vi "Motor.vi"(2 "DESV-IN":bool, 3 "BrickReference in":T1) -> (0 "DESV-OUT":bool, 1 "BrickReference out":T1)   [LabVIEW 2015]
uses:
  <vilib>/NXT/Subs/LVHSConnector.ctl
  <vilib>/NXT/LegoClasses/BrickReference/BrickReference.lvclass
  <vilib>/NXT/Block Support/NXT_OutputPort.ctl
  <vilib>/NXT/Subs/MotorOutput.ctl
  <vilib>/NXT/NXTIO Xnodes/NXTIONodeSubVIs/NXTMotorSteeringOn.vi
  <vilib>/NXT/Dual Mode Library/Sound/Tone.vi
  <vilib>/NXT/NXTIO Xnodes/AddressXNode/NXTIOAddress.xnode
  <vilib>/NXT/NXTIO Xnodes/NXTIOXNode/NXTIO.xnode
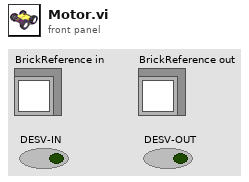
[diagram p1: front panel]
types:
  T1 = typedef "LVHSConnector.ctl" = refnum<class "BrickReference.lvclass">
  T2 = typedef "NXT_OutputPort.ctl" = u8
  T3 = typedef "MotorOutput.ctl" = u8
  T4 = cluster{"PowerLeft":i32, "RotationLeft(Degrees)":i32, "PortLeft":T3}
  T5 = cluster{"PowerRight":i32, "RotationRight(Degrees)":i32, "PortRight":T3}
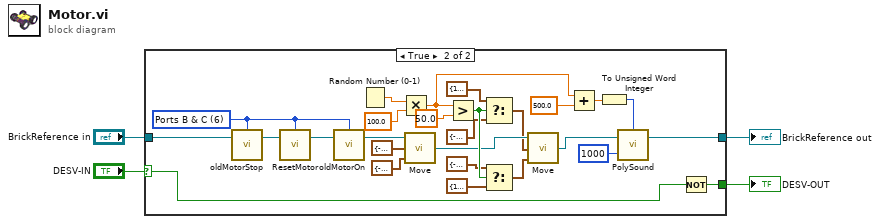
[diagram p0: block diagram]
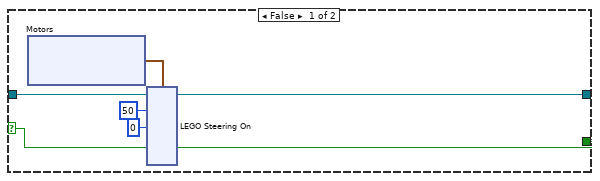
[diagram p2: hidden frame]
diagram:
  n1 = case shown="True" "DESV-IN" {
    selector: "DESV-IN" -> [w6 w22]
    tunnel: "BrickReference in" -> [w10 w46]
    tunnel: [w6 w21] -> w3
    tunnel: [w5 w20] -> w4
    frame False {
      n2 = xnode "Motors"() -> ("Motor"=w9:cluster{"Port":T2, "Port":T2})
      n3 = xnode "LEGO Steering On"("Steering 1"=0, "Power 1"=50, "Motors"=w9, "NXT/EV3"=w10) -> ("NXT/EV3"=w5:T1)
    }
    frame True {
      w43 = T3 6 items=["Port A"=0, "Port B"=1, "Port C"=2, "Ports A & B"=4, "Ports A & C"=5, "Ports B & C"=6, "All Ports"=3] ("Output Port (All Ports)")
      n4 = call <vilib>:"oldMotorStop.vi"("NXT/EV3"=w46, "Output Port (All Ports)"=w43) -> ("NXT/EV3"=w45:T1)  [unwired: 2 in]
      n5 = call <vilib>:"ResetMotor.vi"("NXT/EV3"=w45, "Port (All Ports)"=w43) -> ("NXT/EV3"=w44:T1)  [unwired: 2 in]
      n6 = call <vilib>:"oldMotorOn.vi"("NXT/EV3"=w44, "Output Port (All Ports)"=w43) -> ("NXT/EV3"=w42:T1)  [unwired: 2 in]
      n7 = Random Number (0-1)() -> (number: 0 to 1=w38:dbl)
      n8 = Multiply(x=w38, y=100.0) -> (x*y=w27:dbl)
      n9 = call "Move.vi"("Right"=T4 {"PowerLeft"=-100, "RotationLeft(Degrees)"=-360, "PortLeft"=1} ("Left"), "Left"=T5 {"PowerRight"=-100, "RotationRight(Degrees)"=-360, "PortRight"=2} ("Right"), "BrickReference in"=w42) -> ("BrickReference out"=w31:T1)
      n10 = Greater?(x=w27, y=50.0) -> (0:w36:bool)
      n11 = Select(t=T5 {"PowerRight"=100, "RotationRight(Degrees)"=360, "PortRight"=2} ("Right"), s=w36, f=T5 {"PowerRight"=-100, "RotationRight(Degrees)"=-360, "PortRight"=2} ("Right")) -> (s? t:f=w29:T5)
      n12 = Select(t=T4 {"PowerLeft"=-100, "RotationLeft(Degrees)"=-360, "PortLeft"=1} ("Left"), s=w36, f=T4 {"PowerLeft"=100, "RotationLeft(Degrees)"=360, "PortLeft"=1} ("Left")) -> (s? t:f=w30:T4)
      n13 = call "Move.vi"("Right"=w30, "Left"=w29, "BrickReference in"=w31) -> ("BrickReference out"=w26:T1)
      n14 = Add(x=w27, y=500.0) -> (x+y=w25:dbl)
      n15 = To Unsigned Word Integer(number=w25) -> (unsigned 16bit integer=w24:u16)
      n16 = call-poly <vilib>:"PolySound.vi"("Duration (500 ms)"=u16 1000, "NXT/EV3"=w26, "Tone (440 Hz)"=w24) -> ("NXT/EV3"=w20:T1)  [unwired: 1 in]
      n17 = Not(x=w22) -> (.not. x?=w21:bool)
    }
  }
  "BrickReference out" <- w4
  "DESV-OUT" <- w3
